vi "Update VI Properties.vi"() -> ()   [LabVIEW 2013, in "update vi properties.lvlib"]
uses:
  update vi properties.lvlib
  user action.ctl
  Event Data.ctl
  <vilib>/picture/picture.llb/imagedata.ctl
panel:
  in  "Prompt?":bool
  in  "Adjust all?":bool
  in  "Load":bool
  in  "Error in":errorcluster
  in  "Event Data":T1
  in  "Controls":string[][](table)
  in  "Indicators":string[][](table)
  in  "Help Tag":string
  in  "Help Path":string
  out "Path to VI":string
  in  "VI Description":string
  out "VI Conn Pane":picture
  in  "Select a VI to View/Edit Properties:":i32(listbox)=-1
  in  "Action":T2
  in  "OK":bool
  in  "Cancel":bool
  in  "Apply":bool
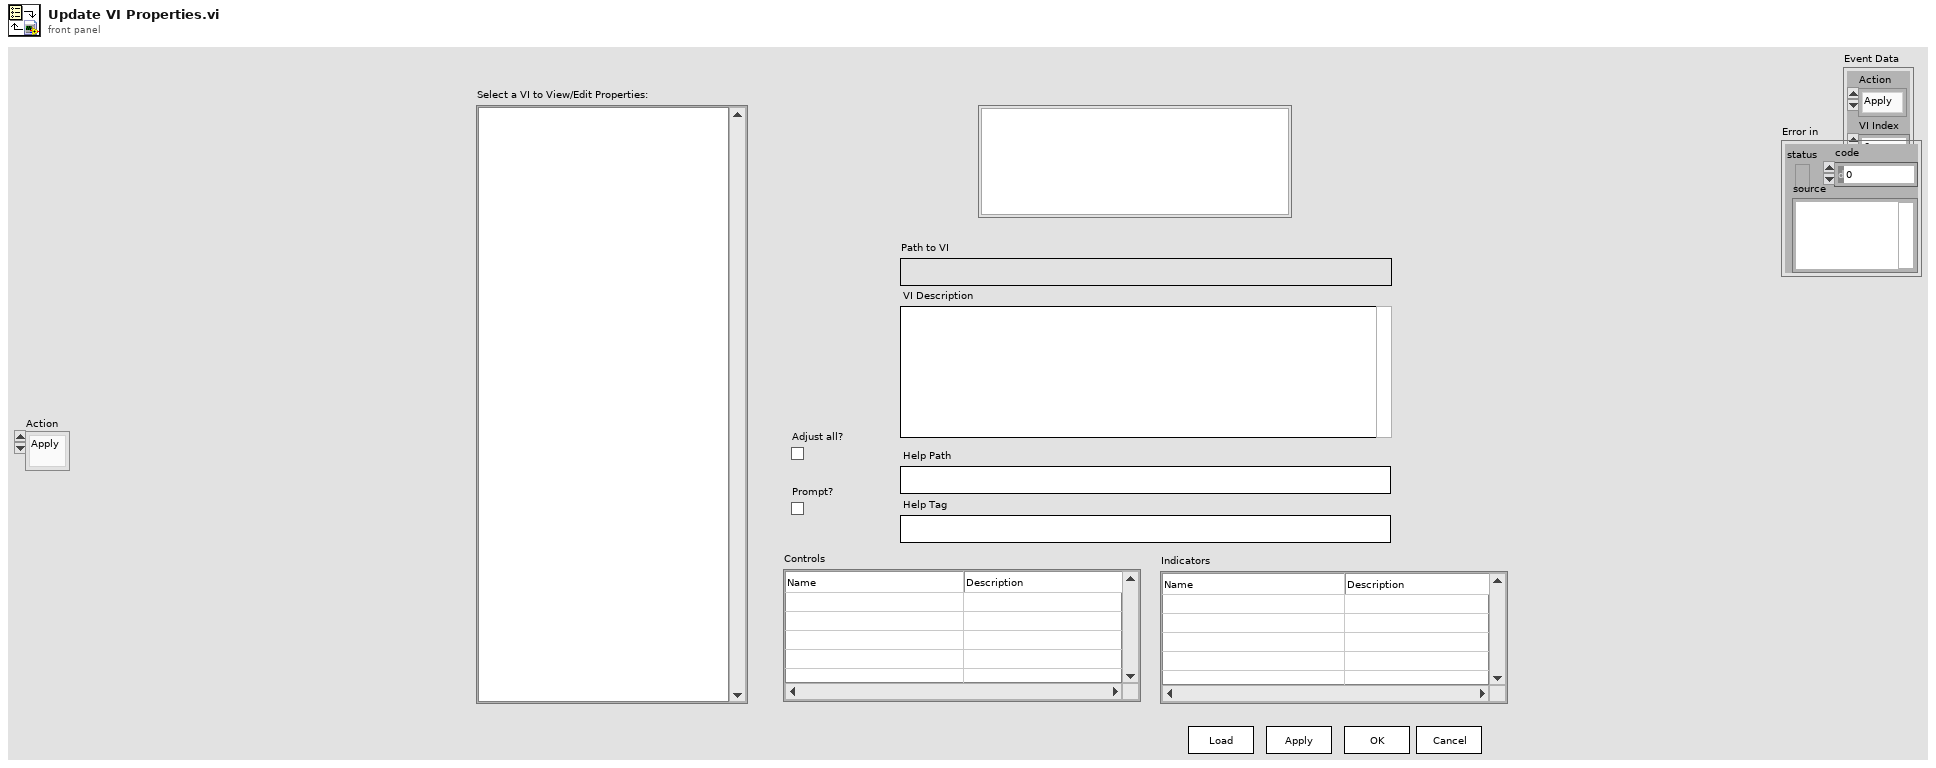
[diagram p1: front panel]
types:
  T1 = typedef "update vi properties.lvlib/Event Data.ctl" = cluster{"Action":T2, "VI Index":i32}
  T2 = typedef "update vi properties.lvlib/user action.ctl" = enum16{"Apply", "Cancel", "VI Selected", "Value Changed", "Load VIs"}
  T3 = typedef "imagedata.ctl" = cluster{"image type":i32, "image depth":i32, "image":u8[], "mask":u8[], "colors":u32[], "Rectangle":cluster{"left":i16, "top":i16, "right":i16, "bottom":i16}}
  T4 = enum32{"invalid VI type", "Standard VI", "Control VI", "Global VI", "Polymorphic VI", "Configuration VI", "SubSystem", "Facade VI", "Method VI", "Statechart Diagram VI"}[]
  T5 = enum32{"invalid VI type", "Standard VI", "Control VI", "Global VI", "Polymorphic VI", "Configuration VI", "SubSystem", "Facade VI", "Method VI", "Statechart Diagram VI"}
  T6 = enum8{"Enabled", "Disabled", "Disabled and Grayed Out"}
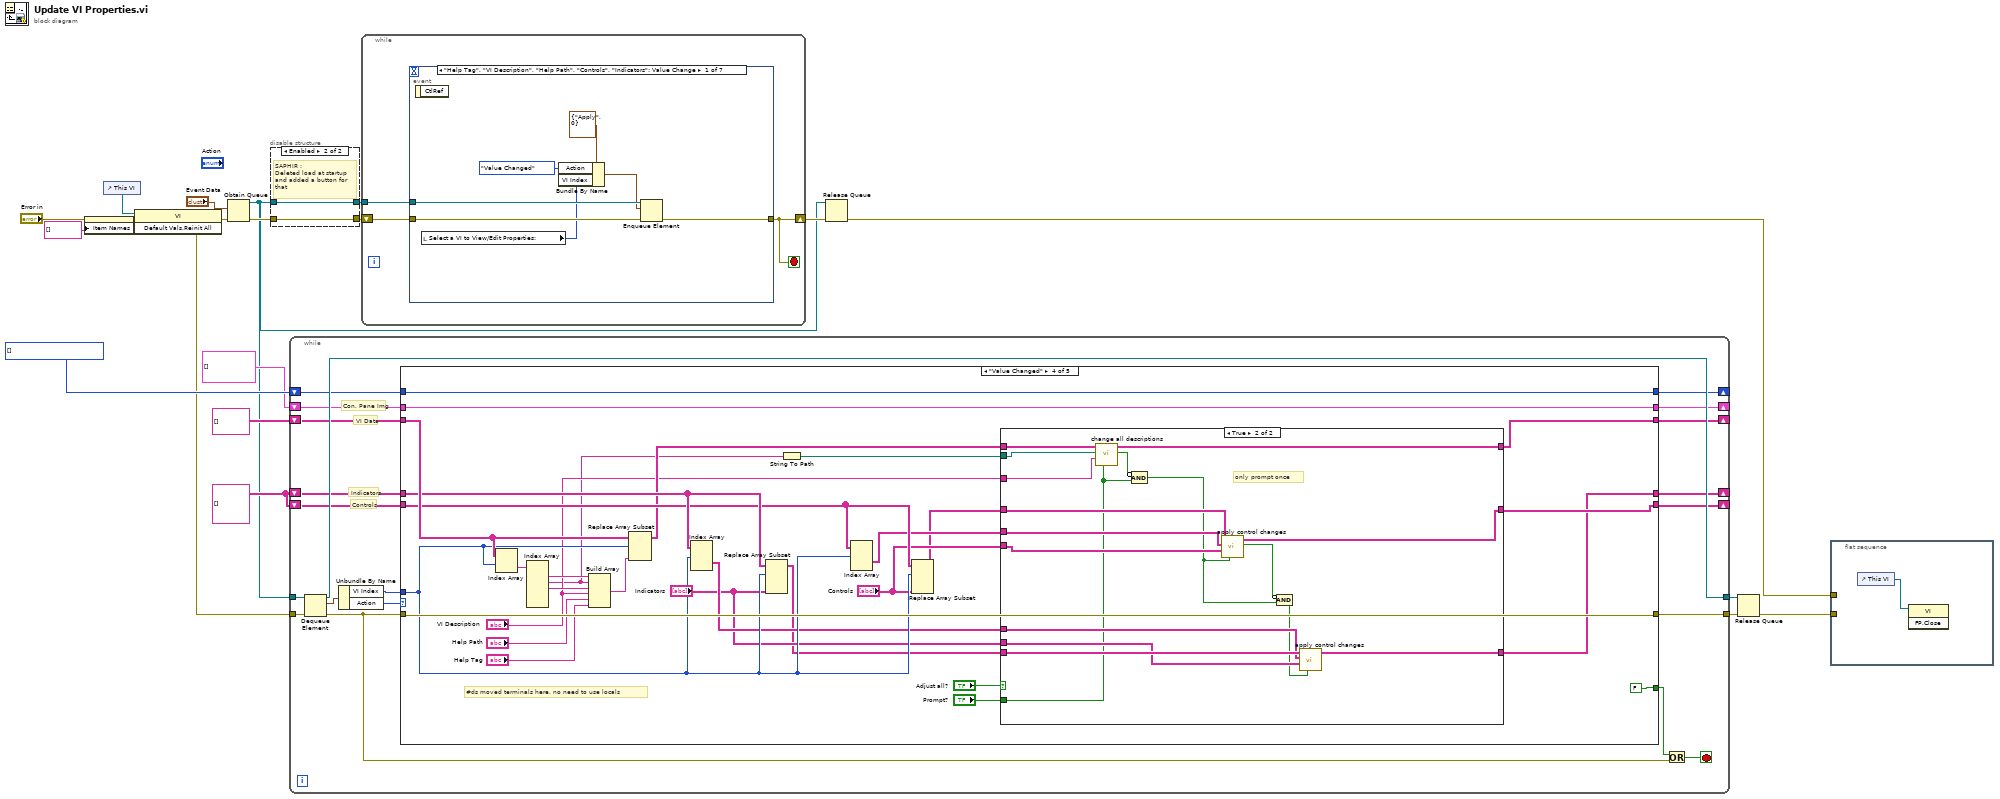
[diagram p0: block diagram]
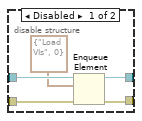
[diagram p2: hidden frame]
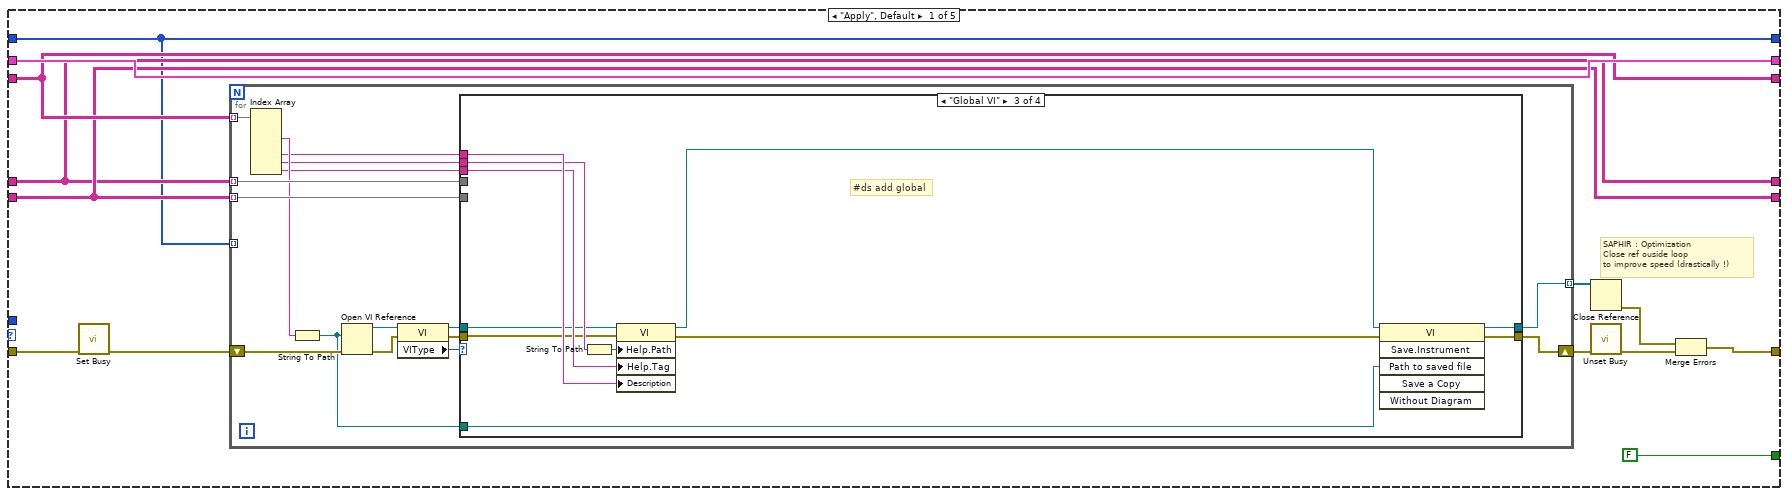
[diagram p3: hidden frame]
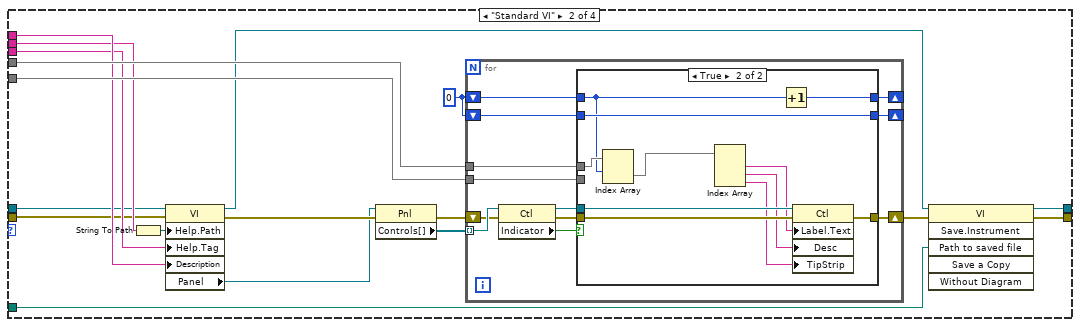
[diagram p5: hidden frame]
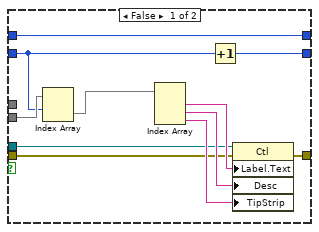
[diagram p6: hidden frame]
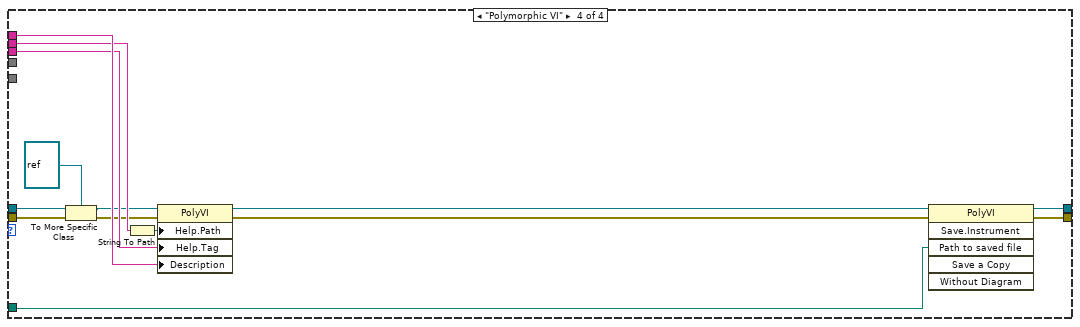
[diagram p7: hidden frame]
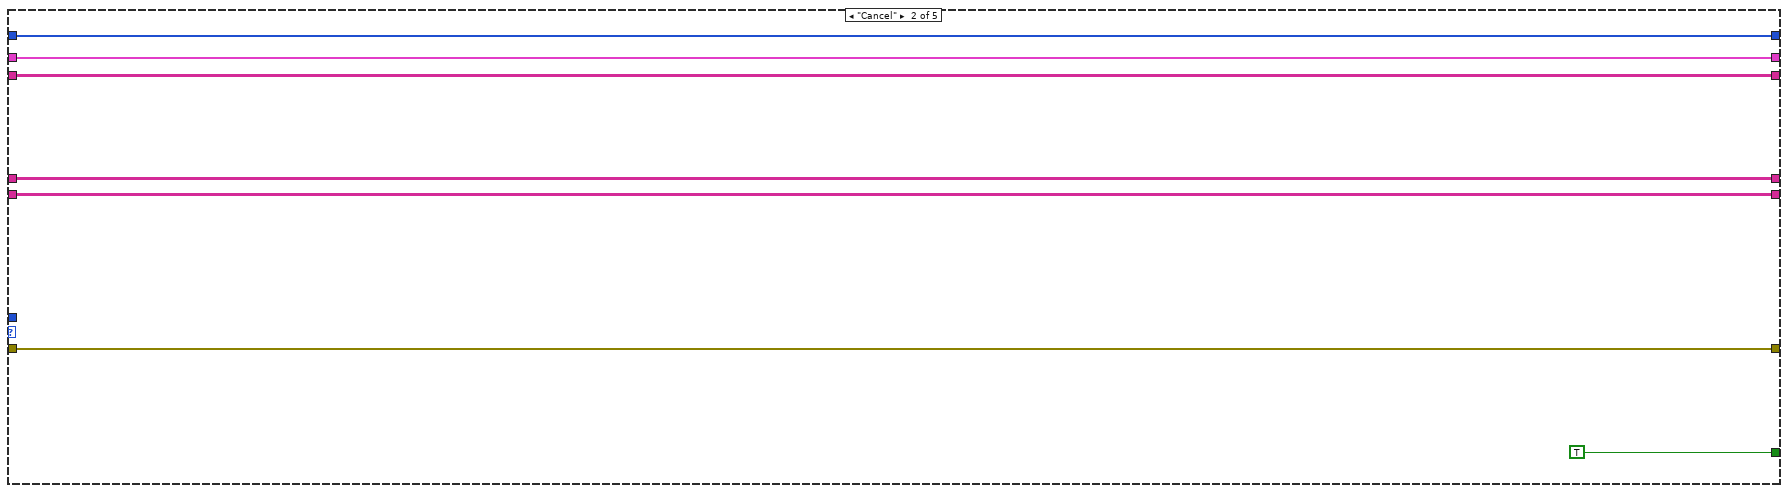
[diagram p8: hidden frame]
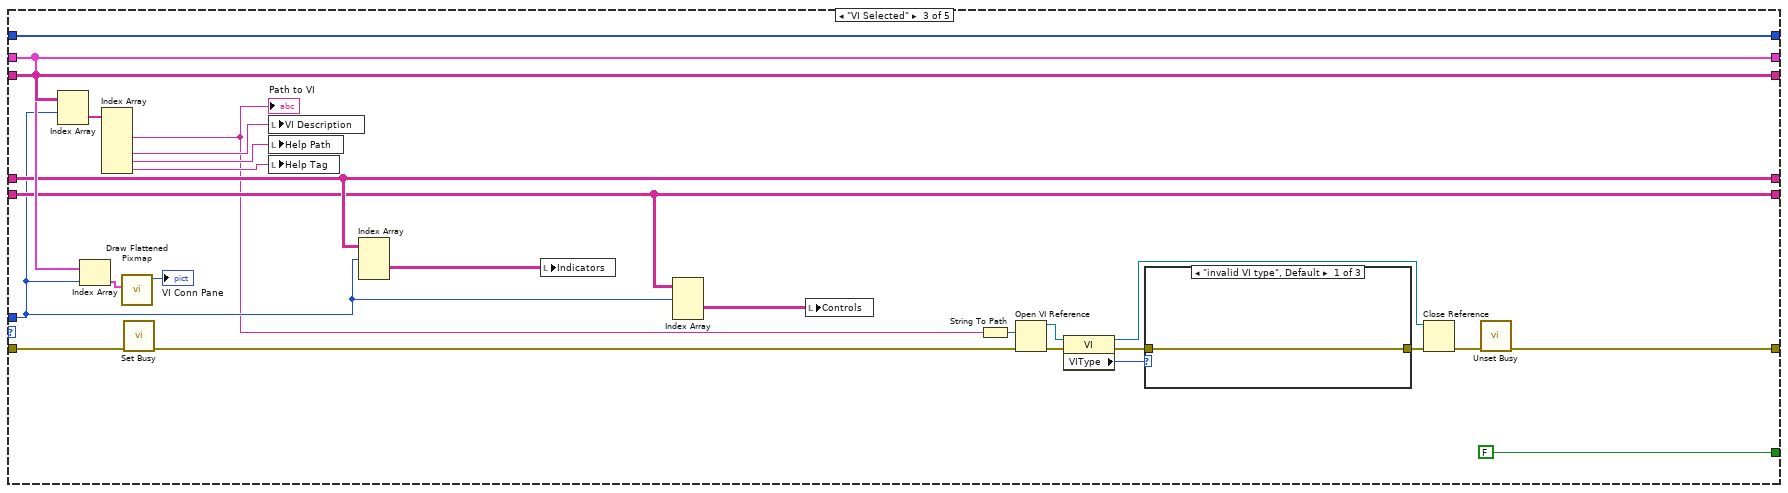
[diagram p9: hidden frame]
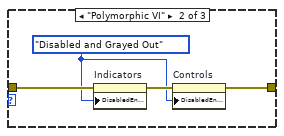
[diagram p10: hidden frame]
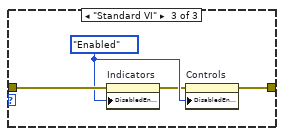
[diagram p11: hidden frame]
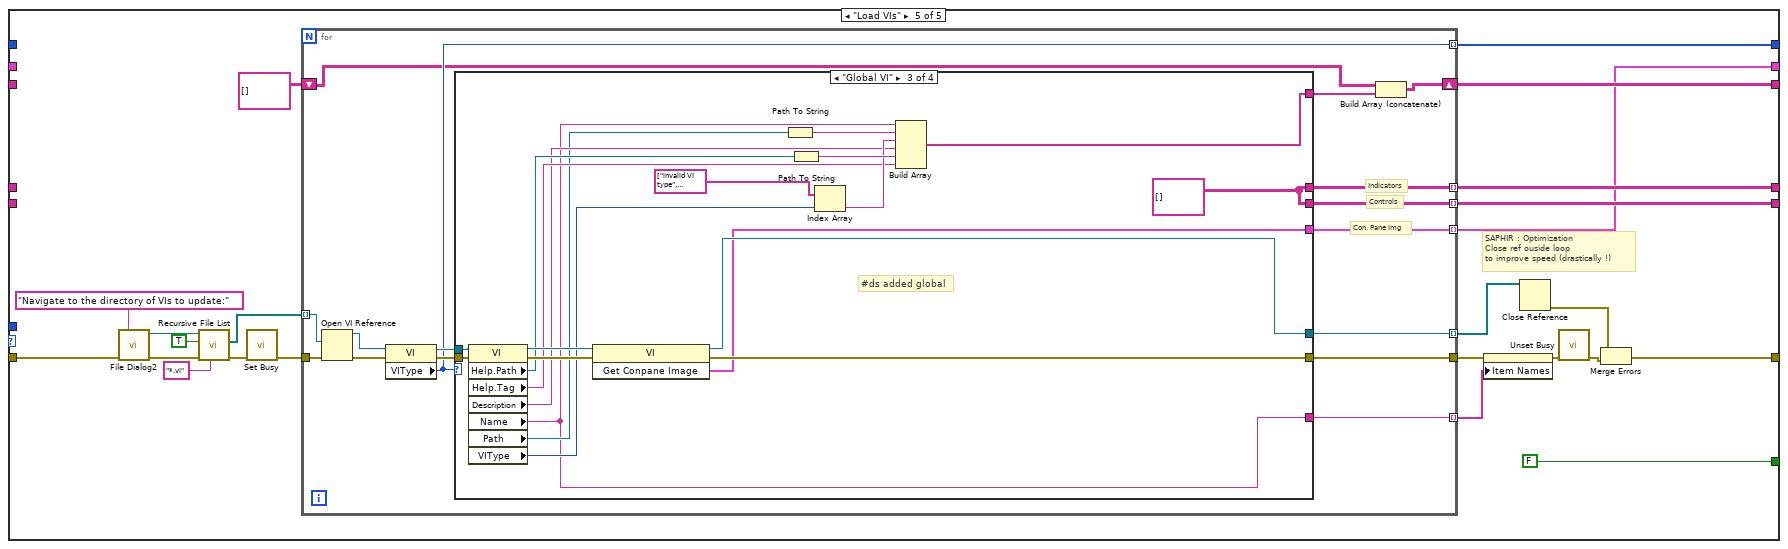
[diagram p13: hidden frame]
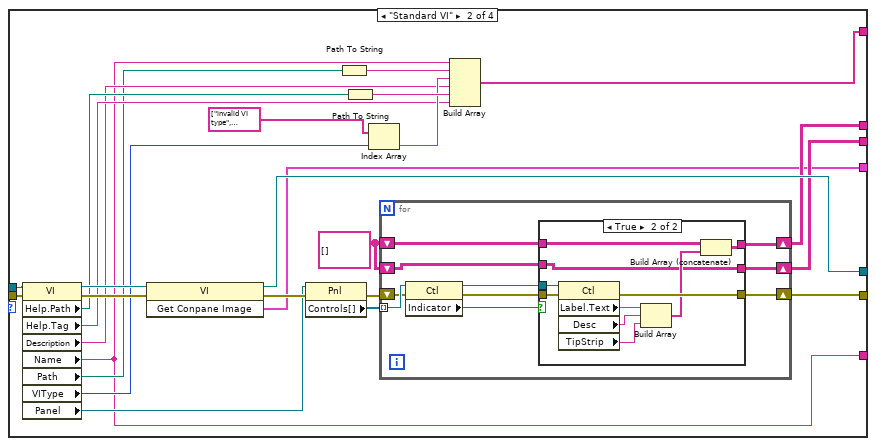
[diagram p15: hidden frame]
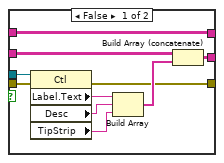
[diagram p16: hidden frame]
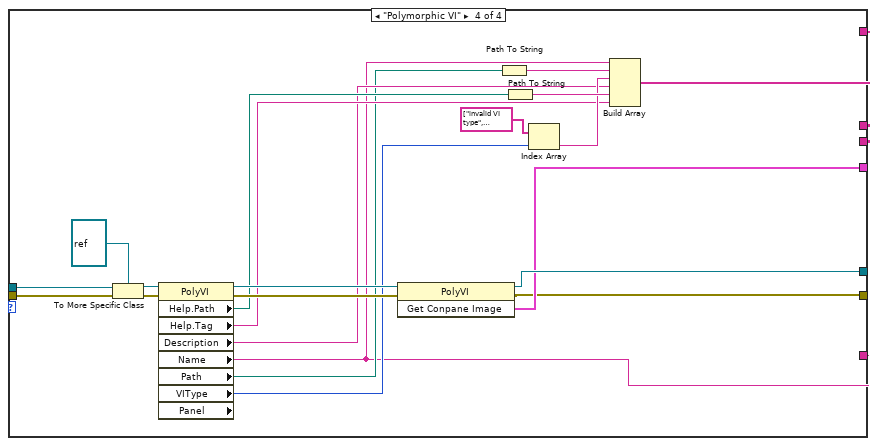
[diagram p17: hidden frame]
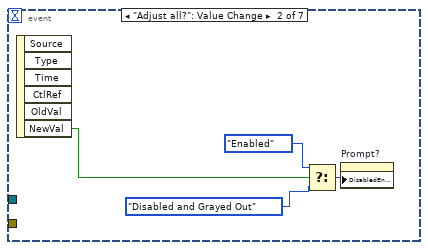
[diagram p18: hidden frame]
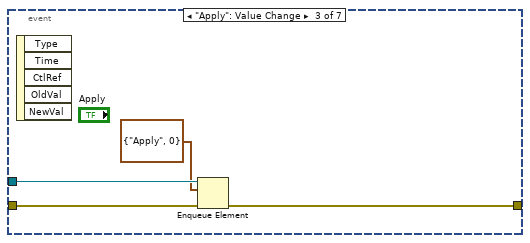
[diagram p19: hidden frame]
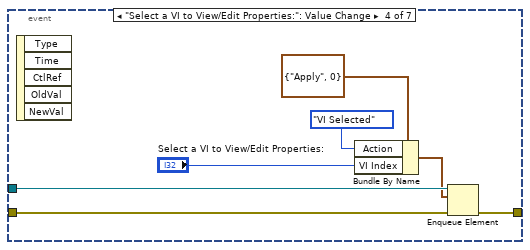
[diagram p20: hidden frame]
diagram:
  w11 = string[][][] []
  w13 = T4 [] items=["invalid VI type", "Standard VI", "Control VI", "Global VI", "Polymorphic VI", "Configuration VI", "SubSystem", "Facade VI", "Method VI", "Statechart Diagram VI"]
  n1 = property on="Select a VI to View/Edit Properties:" class="LstBox (strict)"(error in="Error in", "Item Names"=string[] []) -> (error out=w6:errorcluster)  [unwired: 1 in, 1 out]
  n2 = control-ref of="This VI"() -> (w9:refnum<vi>)
  n3 = invoke class="VI" method="Default Vals.Reinit All"(reference=w9, error in=w6) -> (error out=w8:errorcluster)  [unwired: 1 in, 2 out]
  n4 = Obtain Queue(element data type="Event Data", error in (no error)=w8) -> (queue out=w3:refnum<queue>, error out=w16:errorcluster)  [unwired: 3 in, 1 out]
  n5 = disable-structure shown="Enabled" {
    disable-tunnel: w16 -> [w24 w26]
    disable-tunnel: [w23 w26] -> w15
    disable-tunnel: w3 -> [w22 w25]
    disable-tunnel: [w21 w25] -> w14
    frame Disabled {
      n6 = Enqueue Element(queue=w22, element=T1 {"Action"=enum."Load VIs", "VI Index"=0}, error in (no error)=w24) -> (queue out=w21:refnum<queue>, error out=w23:errorcluster)  [unwired: 1 in, 1 out]
    }
    frame Enabled {
      # "SAPHIR :\nDeleted load at startup\nand added a button for\nthat"
    }
  }
  n7 = while {
    tunnel: w8 -> [w34]
    tunnel: w3 -> [w46]
    tunnel: [w31] -> w19
    tunnel: [w45] -> w18
    shift-right: [w38] -> _
    shift-left: string[][] [] -> [w39]
    shift-right: [w35] -> _
    shift-left: T3[] [] -> [w40]
    shift-right: [w37] -> _
    shift-left: w11 -> [w41]
    shift-right: [w36] -> _
    shift-left: w11 -> [w42]
    shift-right: [w32] -> _
    shift-left: w13 -> [w33]
    stop <- w28 stop-if-true
    # "VI Data"
    # "Controls"
    # "Indicators"
    # "Con. Pane Img"
    n8 = Dequeue Element(queue=w46, error in (no error)=w34) -> (queue out=w45:refnum<queue>, element=w44:T1, error out=w29:errorcluster)  [unwired: 1 in, 1 out]
    n9 = Unbundle By Name(w44) -> ("VI Index"=w43:i32, "Action"=w30:T2)
    n10 = case shown="\"Value Changed\"" w30 {
      tunnel: w29 -> [w58 w160 w180 w225 w265]
      tunnel: [FALSE TRUE FALSE FALSE FALSE] -> w27
      tunnel: [w48 w160 w162 w225 w247] -> w31
      tunnel: w43 -> [_ _ w176 w213 _]
      tunnel: w42 -> [w55 w157 w177 w214 _]
      tunnel: w41 -> [w54 w158 w178 w215 _]
      tunnel: w40 -> [w57 w156 w185 w224 _]
      tunnel: w39 -> [w56 w159 w186 w219 _]
      tunnel: [w56 w159 w186 w202 w259] -> w38
      tunnel: [w54 w158 w178 w204 w256] -> w37
      tunnel: [w55 w157 w177 w205 w255] -> w36
      tunnel: [w57 w156 w185 w224 w254] -> w35
      tunnel: w33 -> [w53 w155 w173 w218 _]
      tunnel: [w53 w155 w173 w218 w258] -> w32
      frame "Apply", Default {
        # "SAPHIR : Optimization\nClose ref ouside loop\nto improve speed (drastically !)"
        n11 = call <vilib>:"Set Busy.vi"("error in (no error)"=w58) -> ("error out"=w52:errorcluster)  [unwired: 9 in, 1 out]
        n12 = for {
          shift-right: [w61] -> w51
          shift-left: w52 -> [w74]
          tunnel: w56 -> [w75] mode=indexing
          tunnel: w55 -> [w72] mode=indexing
          tunnel: w54 -> [w73] mode=indexing
          tunnel: w53 -> [_] mode=indexing
          tunnel: [w60] -> w49 mode=indexing
          n13 = Index Array(array=w75) -> (element #2=w71:string, element #4=w70:string, element #5=w68:string, element #6=w69:string)  [unwired: 6 in, 2 out]
          n14 = String To Path(string=w71) -> (path=w67:path)
          n15 = Open VI Reference(vi path=w67, error in (no error)=w74) -> (vi reference=w66:refnum<vi>, error out=w63:errorcluster)  [unwired: 4 in]
          n16 = property class="VI"(reference=w66, error in=w63) -> (reference out=w65:refnum<vi>, error out=w64:errorcluster, "VIType"=w62:T5)
          n17 = case shown="\"Global VI\"" w62 {
            tunnel: [w76 w95 w140 w154] -> w60
            tunnel: [w77 w94 w139 w153] -> w61
            tunnel: w73 -> [_ w93 _ _]
            tunnel: w72 -> [_ w92 _ _]
            tunnel: w65 -> [w76 w79 w131 w146]
            tunnel: w64 -> [w77 w78 w130 w145]
            tunnel: w70 -> [_ w91 w138 w152]
            tunnel: w69 -> [_ w90 w137 w151]
            tunnel: w68 -> [_ w88 w135 w149]
            tunnel: w67 -> [_ w87 w134 w148]
            frame "invalid VI type", Default {
            }
            frame "Standard VI" {
              w80 = 0
              n18 = String To Path(string=w88) -> (path=w89:path)
              n19 = property class="VI"(reference=w79, error in=w78, "Help.Path"=w89, "Help.Tag"=w90, "Description"=w91) -> (reference out=w83:refnum<vi>, error out=w86:errorcluster, "Panel"=w85:refnum<vi>)
              n20 = property class="Pnl"(reference=w85, error in=w86) -> (error out=w81:errorcluster, "Controls[]"=w82:refnum<vi>[])  [unwired: 1 out]
              n21 = for {
                tunnel: w82 -> [w107] mode=indexing
                shift-right: [w96] -> w84
                shift-left: w81 -> [w106]
                tunnel: w93 -> [w99]
                tunnel: w92 -> [w98]
                shift-right: [w101] -> _
                shift-left: w80 -> [w103]
                shift-right: [w100] -> _
                shift-left: w80 -> [w102]
                n22 = property class="Ctl"(reference=w107, error in=w106) -> (reference out=w97:refnum<vi>, error out=w104:errorcluster, "Indicator"=w105:bool)
                n23 = case shown="True" w105 {
                  tunnel: w104 -> [w109 w123]
                  tunnel: w103 -> [w117 w126]
                  tunnel: w102 -> [w108 w128]
                  tunnel: [w117 w129] -> w101
                  tunnel: [w118 w128] -> w100
                  tunnel: w99 -> [_ w127]
                  tunnel: w98 -> [w112 _]
                  tunnel: w97 -> [w110 w124]
                  tunnel: [w113 w122] -> w96
                  frame False {
                    n24 = Index Array(array=w112, index (row)=w108) -> (element=w116:string[])  [unwired: 1 in]
                    n25 = Index Array(array=w116) -> (element #1=w115:string, element #2=w114:string, element #3=w111:string)  [unwired: 3 in]
                    n26 = Increment(x=w108) -> (x+1=w118:i32)
                    n27 = property class="Ctl"(reference=w110, error in=w109, "Label.Text"=w115, "Desc"=w114, "TipStrip"=w111) -> (error out=w113:errorcluster)  [unwired: 1 out]
                  }
                  frame True {
                    n28 = Index Array(array=w127, index (row)=w126) -> (element=w125:string[])  [unwired: 1 in]
                    n29 = Index Array(array=w125) -> (element #1=w121:string, element #2=w120:string, element #3=w119:string)  [unwired: 3 in]
                    n30 = Increment(x=w126) -> (x+1=w129:i32)
                    n31 = property class="Ctl"(reference=w124, error in=w123, "Label.Text"=w121, "Desc"=w120, "TipStrip"=w119) -> (error out=w122:errorcluster)  [unwired: 1 out]
                  }
                }
              }
              n32 = invoke class="VI" method="Save.Instrument"(reference=w83, error in=w84, "Path to saved file"=w87) -> (reference out=w95:refnum<vi>, error out=w94:errorcluster)  [unwired: 3 in, 4 out]
            }
            frame "Global VI" {
              # "#ds add global"
              n33 = String To Path(string=w135) -> (path=w136:path)
              n34 = property class="VI"(reference=w131, error in=w130, "Help.Path"=w136, "Help.Tag"=w137, "Description"=w138) -> (reference out=w132:refnum<vi>, error out=w133:errorcluster)
              n35 = invoke class="VI" method="Save.Instrument"(reference=w132, error in=w133, "Path to saved file"=w134) -> (reference out=w140:refnum<vi>, error out=w139:errorcluster)  [unwired: 3 in, 4 out]
            }
            frame "Polymorphic VI" {
              n36 = To More Specific Class(target class=refnum<vi> refnum, reference=w146, error in=w145) -> (specific class reference=w144:refnum<vi>, error out=w143:errorcluster)
              n37 = String To Path(string=w149) -> (path=w150:path)
              n38 = property class="PolyVI"(reference=w144, error in=w143, "Help.Path"=w150, "Help.Tag"=w151, "Description"=w152) -> (reference out=w142:refnum<vi>, error out=w141:errorcluster)
              n39 = invoke class="PolyVI" method="Save.Instrument"(reference=w142, error in=w141, "Path to saved file"=w148) -> (reference out=w154:refnum<vi>, error out=w153:errorcluster)  [unwired: 3 in, 4 out]
            }
          }
        }
        n40 = Close Reference(reference=w49) -> (error out=w47:errorcluster)  [unwired: 1 in]
        n41 = call <vilib>:"Unset Busy.vi"("error in (no error)"=w51) -> ("error out"=w50:errorcluster)  [unwired: 10 in]
        n42 = Merge Errors(w47, w50) -> (w48:errorcluster)
      }
      frame "Cancel" {
      }
      frame "VI Selected" {
        n43 = Index Array(array=w186, index (row)=w176) -> (element=w184:string[])  [unwired: 1 in]
        n44 = Index Array(array=w185, index=w176) -> (element=w187:T3)
        n45 = Index Array(array=w184) -> (element #2=w172:string, element #4=w183:string, element #5=w182:string, element #6=w181:string)  [unwired: 6 in, 2 out]
        "Path to VI" <- w172
        n46 = call <vilib>:"Draw Flattened Pixmap.vi"("image data"=w187) -> ("new picture"=→"VI Conn Pane":picture)  [unwired: 8 in]
        n47 = call <vilib>:"Set Busy.vi"("error in (no error)"=w180) -> ("error out"=w163:errorcluster)  [unwired: 9 in, 1 out]
        n48 = local write "VI Description"(w183) -> ()
        n49 = local write "Help Path"(w182) -> ()
        n50 = local write "Help Tag"(w181) -> ()
        n51 = Index Array(array=w178, index (dim 0)=w176) -> (element=w174:string[][])  [unwired: 2 in]
        n52 = local write "Indicators"(w174) -> ()
        n53 = Index Array(array=w177, index (dim 0)=w176) -> (element=w175:string[][])  [unwired: 2 in]
        n54 = local write "Controls"(w175) -> ()
        n55 = String To Path(string=w172) -> (path=w171:path)
        n56 = Open VI Reference(vi path=w171, error in (no error)=w163) -> (vi reference=w170:refnum<vi>, error out=w169:errorcluster)  [unwired: 4 in]
        n57 = property class="VI"(reference=w170, error in=w169) -> (reference out=w164:refnum<vi>, error out=w167:errorcluster, "VIType"=w168:T5)
        n58 = case shown="\"invalid VI type\", Default" w168 {
          tunnel: w167 -> [w189 w192 w197]
          tunnel: [w189 w191 w194] -> w166
          frame "invalid VI type", Default {
          }
          frame "Polymorphic VI" {
            w190 = T6."Disabled and Grayed Out" ("Disabled")
            n59 = property on="Indicators" class="Tbl (strict)"(error in=w192, "DisabledEnum"=w190) -> (error out=w193:errorcluster)  [unwired: 1 in, 1 out]
            n60 = property on="Controls" class="Tbl (strict)"(error in=w193, "DisabledEnum"=w190) -> (error out=w191:errorcluster)  [unwired: 1 in, 1 out]
          }
          frame "Standard VI" {
            w196 = T6."Enabled" ("Disabled")
            n61 = property on="Indicators" class="Tbl (strict)"(error in=w197, "DisabledEnum"=w196) -> (error out=w195:errorcluster)  [unwired: 1 in, 1 out]
            n62 = property on="Controls" class="Tbl (strict)"(error in=w195, "DisabledEnum"=w196) -> (error out=w194:errorcluster)  [unwired: 1 in, 1 out]
          }
        }
        n63 = Close Reference(reference=w164, error in (no error)=w166) -> (error out=w165:errorcluster)
        n64 = call <vilib>:"Unset Busy.vi"("error in (no error)"=w165) -> ("error out"=w162:errorcluster)  [unwired: 10 in]
      }
      frame "Value Changed" {
        # "#ds moved terminals here, no need to use locals"
        n65 = Index Array(array=w219, index (row)=w213) -> (element=w223:string[])  [unwired: 1 in]
        n66 = Index Array(array=w223) -> (element #1=w222:string, element #2=w199:string, element #3=w221:string)  [unwired: 6 in, 3 out]
        n67 = Build Array(w222, w199, w221, "VI Description", "Help Path", "Help Tag") -> (w220:string[])
        n68 = Replace Array Subset(array=w219, new element=w220, index (row)=w213) -> (w201:string[][])  [unwired: 1 in]
        n69 = Index Array(array=w215, index (dim 0)=w213) -> (element=w208:string[][])  [unwired: 2 in]
        n70 = Replace Array Subset(array=w215, new element="Indicators", index (dim 0)=w213) -> (w203:string[][][])  [unwired: 2 in]
        n71 = String To Path(string=w199) -> (path=w198:path)
        n72 = Index Array(array=w214, index (dim 0)=w213) -> (element=w209:string[][])  [unwired: 2 in]
        n73 = Replace Array Subset(array=w214, new element="Controls", index (dim 0)=w213) -> (w206:string[][][])  [unwired: 2 in]
        n74 = case shown="True" "Adjust all?" {
          tunnel: "Prompt?" -> [_ w234]
          tunnel: "Controls" -> [_ w240]
          tunnel: w209 -> [_ w241]
          tunnel: w208 -> [_ w238]
          tunnel: "Indicators" -> [_ w237]
          tunnel: w206 -> [w229 w243]
          tunnel: [w229 w242] -> w205
          tunnel: w203 -> [w228 w239]
          tunnel: [w228 w236] -> w204
          tunnel: [w227 w246] -> w202
          tunnel: w201 -> [w227 w245]
          tunnel: "VI Description" -> [_ w235]
          tunnel: w198 -> [_ w244]
          frame False {
          }
          frame True {
            # "only prompt once"
            n75 = call "change all descriptions.vi"("Prompt?"=w234, "new"=w235, "Path"=w244, "dataset in"=w245) -> ("adjust all"=w233:bool, "dataset out"=w246:string[][])  [unwired: 6 in]
            n76 = Compound Arithmetic op=AND(invert w233, w234) -> (w231:bool)
            n77 = call "apply control changes.vi"("Prompt?"=w231, "new"=w240, "old"=w241, "dataset in"=w243) -> ("adjust all?"=w232:bool, "dataset out"=w242:string[][][])  [unwired: 6 in]
            n78 = Compound Arithmetic op=AND(invert w232, w231) -> (w230:bool)
            n79 = call "apply control changes.vi"("Prompt?"=w230, "new"=w237, "old"=w238, "dataset in"=w239) -> ("dataset out"=w236:string[][][])  [unwired: 6 in, 1 out]
          }
        }
      }
      frame "Load VIs" {
        # "SAPHIR : Optimization\nClose ref ouside loop\nto improve speed (drastically !)"
        n80 = call "File Dialog2"("prompt"="Navigate to the directory of VIs to update:", "error in"=w265) -> ("selected path"=w267:path, "error out"=w268:errorcluster)  [unwired: 10 in, 2 out]
        n81 = call <vilib>:"Recursive File List.vi"("pattern"="*.vi", "error in (no error)"=w268, "Treat LLBs as Folders?"=TRUE, "Folder Path"=w267) -> ("error out"=w263:errorcluster, "All Files in Dir"=w261:path[])  [unwired: 3 in, 3 out]
        n82 = call <vilib>:"Set Busy.vi"("error in (no error)"=w263) -> ("error out"=w262:errorcluster)  [unwired: 9 in, 1 out]
        n83 = for {
          tunnel: w262 -> [w283]
          tunnel: w261 -> [w282] mode=indexing
          shift-right: [w276] -> w259
          shift-left: string[][] [] -> [w278]
          tunnel: [w279] -> w258 mode=indexing
          tunnel: [w275] -> w257 mode=indexing
          tunnel: [w274] -> w256 mode=indexing
          tunnel: [w273] -> w255 mode=indexing
          tunnel: [w272] -> w254 mode=indexing
          tunnel: [w271] -> w253
          tunnel: [w270] -> w250 mode=indexing
          # "Controls"
          # "Indicators"
          # "Con. Pane Img"
          n84 = Open VI Reference(vi path=w282, error in (no error)=w283) -> (vi reference=w285:refnum<vi>, error out=w284:errorcluster)  [unwired: 4 in]
          n85 = property class="VI"(reference=w285, error in=w284) -> (reference out=w280:refnum<vi>, error out=w281:errorcluster, "VIType"=w279:T5)
          n86 = case shown="\"Global VI\"" w279 {
            tunnel: w281 -> [w287 w316 w365 w371]
            tunnel: w280 -> [w286 w315 w364 w369]
            tunnel: [string[] ["Invalid VI type"] w297 w349 w374] -> w277
            tunnel: ["" ("Name") w296 w348 w373] -> w275
            tunnel: [w289 w309 w347 w366] -> w274
            tunnel: [w289 w308 w347 w366] -> w273
            tunnel: [T3 {"image type"=0, "image depth"=0, "image"=[], "mask"=[], "colors"=[], "Rectangle"={"left"=0, "top"=0, "right"=0, "bottom"=0}} ("Get Conpane Image") w307 w359 w384] -> w272
            tunnel: [w287 w295 w361 w367] -> w271
            tunnel: [w286 w310 w360 w385] -> w270
            frame "invalid VI type", Default {
              w289 = string[][] []
            }
            frame "Standard VI" {
              w292 = string[][] []
              n87 = property class="VI"(reference=w315, error in=w316) -> (reference out=w314:refnum<vi>, error out=w313:errorcluster, "Help.Path"=w302:path, "Help.Tag"=w301:string, "Description"=w300:string, "Name"=w296:string, "Path"=w299:path, "VIType"=w298:T5, "Panel"=w311:refnum<vi>)
              n88 = invoke class="VI" method="Get Conpane Image"(reference=w314, error in=w313) -> (reference out=w310:refnum<vi>, error out=w312:errorcluster, "Get Conpane Image"=w307:T3)  [unwired: 1 in]
              n89 = property class="Pnl"(reference=w311, error in=w312) -> (error out=w293:errorcluster, "Controls[]"=w294:refnum<vi>[])  [unwired: 1 out]
              n90 = Path To String(path=w299) -> (string=w304:string)
              n91 = Path To String(path=w302) -> (string=w306:string)
              n92 = Index Array(array=string[] ["invalid VI type", "Standard VI", "Control VI", "Global VI", "Polymorphic VI", "Configuration VI", "SubSystem", "Facade VI", "Method VI", "Statechart Diagram VI"] ("Strings []"), index=w298) -> (element=w305:string)
              n93 = for {
                tunnel: w294 -> [w326] mode=indexing
                shift-right: [w321] -> w295
                shift-left: w293 -> [w325]
                shift-right: [w320] -> w309
                shift-left: w292 -> [w319]
                shift-right: [w318] -> w308
                shift-left: w292 -> [w317]
                n94 = property class="Ctl"(reference=w326, error in=w325) -> (reference out=w323:refnum<vi>, error out=w322:errorcluster, "Indicator"=w324:bool)
                n95 = case shown="True" w324 {
                  tunnel: w323 -> [w331 w346]
                  tunnel: w322 -> [w332 w345]
                  tunnel: [w330 w344] -> w321
                  tunnel: [w327 w338] -> w320
                  tunnel: w319 -> [w327 w340]
                  tunnel: [w329 w337] -> w318
                  tunnel: w317 -> [w328 w337]
                  frame False {
                    n96 = property class="Ctl"(reference=w331, error in=w332) -> (error out=w330:errorcluster, "Label.Text"=w336:string, "Desc"=w335:string, "TipStrip"=w334:string)  [unwired: 1 out]
                    n97 = Build Array(w336, w335, w334) -> (w333:string[])
                    n98 = Build Array (concatenate)(w328, w333) -> (w329:string[][])
                  }
                  frame True {
                    n99 = property class="Ctl"(reference=w346, error in=w345) -> (error out=w344:errorcluster, "Label.Text"=w343:string, "Desc"=w342:string, "TipStrip"=w341:string)  [unwired: 1 out]
                    n100 = Build Array(w343, w342, w341) -> (w339:string[])
                    n101 = Build Array (concatenate)(w340, w339) -> (w338:string[][])
                  }
                }
              }
              n102 = Build Array(w296, w304, w305, w300, w306, w301) -> (w297:string[])
            }
            frame "Global VI" {
              w347 = string[][] []
              # "#ds added global"
              n103 = property class="VI"(reference=w364, error in=w365) -> (reference out=w363:refnum<vi>, error out=w362:errorcluster, "Help.Path"=w354:path, "Help.Tag"=w353:string, "Description"=w352:string, "Name"=w348:string, "Path"=w351:path, "VIType"=w350:T5)
              n104 = invoke class="VI" method="Get Conpane Image"(reference=w363, error in=w362) -> (reference out=w360:refnum<vi>, error out=w361:errorcluster, "Get Conpane Image"=w359:T3)  [unwired: 1 in]
              n105 = Path To String(path=w351) -> (string=w356:string)
              n106 = Path To String(path=w354) -> (string=w358:string)
              n107 = Index Array(array=string[] ["invalid VI type", "Standard VI", "Control VI", "Global VI", "Polymorphic VI", "Configuration VI", "SubSystem", "Facade VI", "Method VI", "Statechart Diagram VI"] ("Strings []"), index=w350) -> (element=w357:string)
              n108 = Build Array(w348, w356, w357, w352, w358, w353) -> (w349:string[])
            }
            frame "Polymorphic VI" {
              w366 = string[][] []
              n109 = To More Specific Class(target class=refnum<vi> refnum, reference=w369, error in=w371) -> (specific class reference=w368:refnum<vi>, error out=w370:errorcluster)
              n110 = property class="PolyVI" props=["Help.Path", "Help.Tag", "Description", "Name", "Path", "VIType", "Panel"](reference=w368, error in=w370) -> (reference out=w387:refnum<vi>, error out=w386:errorcluster, "Help.Path"=w379:path, "Help.Tag"=w378:string, "Description"=w377:string, "Name"=w373:string, "Path"=w376:path, "VIType"=w375:T5)  [unwired: 1 out]
              n111 = invoke class="PolyVI" method="Get Conpane Image"(reference=w387, error in=w386) -> (reference out=w385:refnum<vi>, error out=w367:errorcluster, "Get Conpane Image"=w384:T3)  [unwired: 1 in]
              n112 = Path To String(path=w376) -> (string=w381:string)
              n113 = Path To String(path=w379) -> (string=w383:string)
              n114 = Index Array(array=string[] ["invalid VI type", "Standard VI", "Control VI", "Global VI", "Polymorphic VI", "Configuration VI", "SubSystem", "Facade VI", "Method VI", "Statechart Diagram VI"] ("Strings []"), index=w375) -> (element=w382:string)
              n115 = Build Array(w373, w381, w382, w377, w383, w378) -> (w374:string[])
            }
          }
          n116 = Build Array (concatenate)(w278, w277) -> (w276:string[][])
        }
        n117 = property on="Select a VI to View/Edit Properties:" class="LstBox (strict)"(error in=w253, "Item Names"=w257) -> (error out=w251:errorcluster)  [unwired: 1 in, 1 out]
        n118 = Close Reference(reference=w250) -> (error out=w249:errorcluster)  [unwired: 1 in]
        n119 = call <vilib>:"Unset Busy.vi"("error in (no error)"=w251) -> ("error out"=w248:errorcluster)  [unwired: 10 in]
        n120 = Merge Errors(w249, w248) -> (w247:errorcluster)
      }
    }
    n121 = Or(x=w27, y=w29) -> (x .or. y?=w28:bool)
  }
  n122 = while {
    shift-right: [w388] -> w4
    shift-left: w15 -> [w389]
    tunnel: w14 -> [w390]
    stop <- w388 stop-if-true
    n123 = event shown="[0] \"Help Tag\", \"VI Description\", \"Help Path\", \"Controls\", \"Indicators\": Value Change" {
      selector: _ -> [_ _ _ _ _ _ _]
      dyn-events: _ -> [_ _ _ _ _ _ _]
      timeout: _ -> [_ _ _ _ _ _ _]
      tunnel: w390 -> [w397 _ w405 w412 w416 w422 w426]
      tunnel: w389 -> [w396 _ w404 w411 w415 w423 w425]
      tunnel: [w395 _ w403 w407 w414 w419 w424] -> w388
      event "Help Tag", "VI Description", "Help Path", "Controls", "Indicators": Value Change {
        n124 = event-data() -> ()  [unwired: 1 in, 1 out]
        n125 = local read "Select a VI to View/Edit Properties:"() -> (w392:i32)
        n126 = Bundle By Name(cluster=T1 {"Action"=enum."Apply", "VI Index"=0} ("element"), "Action"=user_action."Value Changed", "VI Index"=w392) -> (w391:T1)
        n127 = Enqueue Element(queue=w397, element=w391, error in (no error)=w396) -> (error out=w395:errorcluster)  [unwired: 1 in, 2 out]
      }
      event "Adjust all?": Value Change {
        n128 = event-data() -> ("NewVal"=w398:bool)  [unwired: 1 in, 5 out]
        n129 = Select(t=T6."Enabled" ("Disabled"), s=w398, f=T6."Disabled and Grayed Out" ("Disabled")) -> (s? t:f=w401:T6)
        n130 = property on="Prompt?" class="Bool (strict)"("DisabledEnum"=w401) -> ()  [unwired: 2 in, 2 out]
      }
      event "Apply": Value Change {
        n131 = event-data() -> ()  [unwired: 1 in, 5 out]
        n132 = Enqueue Element(queue=w405, element=T1 {"Action"=enum."Apply", "VI Index"=0}, error in (no error)=w404) -> (error out=w403:errorcluster)  [unwired: 1 in, 2 out]
      }
      event "Select a VI to View/Edit Properties:": Value Change {
        n133 = event-data() -> ()  [unwired: 1 in, 5 out]
        n134 = Bundle By Name(cluster=T1 {"Action"=enum."Apply", "VI Index"=0} ("element"), "Action"=user_action."VI Selected", "VI Index"="Select a VI to View/Edit Properties:") -> (w408:T1)
        n135 = Enqueue Element(queue=w412, element=w408, error in (no error)=w411) -> (error out=w407:errorcluster)  [unwired: 1 in, 2 out]
      }
      event "Cancel": Value Change {
        n136 = event-data() -> ()  [unwired: 1 in, 5 out]
        n137 = Enqueue Element(queue=w416, element=T1 {"Action"=enum."Cancel", "VI Index"=0}, error in (no error)=w415) -> (error out=w414:errorcluster)  [unwired: 1 in, 2 out]
      }
      event "OK": Value Change {
        (unwired) FALSE ("Cancel")
        n138 = event-data() -> ()  [unwired: 1 in, 5 out]
        n139 = Enqueue Element(queue=w422, element=T1 {"Action"=enum."Apply", "VI Index"=0}, error in (no error)=w423) -> (queue out=w420:refnum<queue>, error out=w421:errorcluster)  [unwired: 1 in, 1 out]
        n140 = Enqueue Element(queue=w420, element=T1 {"Action"=enum."Cancel", "VI Index"=0}, error in (no error)=w421) -> (error out=w419:errorcluster)  [unwired: 1 in, 2 out]
      }
      event "Load": Value Change {
        n141 = event-data() -> ()  [unwired: 1 in, 5 out]
        n142 = Enqueue Element(queue=w426, element=T1 {"Action"=enum."Load VIs", "VI Index"=0}, error in (no error)=w425) -> (error out=w424:errorcluster)  [unwired: 1 in, 2 out]
      }
    }
  }
  n143 = Release Queue(queue=w3, error in (no error)=w4) -> (error out=w1:errorcluster)  [unwired: 1 in, 2 out]
  n144 = Release Queue(queue=w18, error in (no error)=w19) -> (error out=w2:errorcluster)  [unwired: 1 in, 2 out]
  n145 = flat-sequence {
    tunnel: w2 -> [_]
    tunnel: w1 -> [_]
    frame #0 {
      n146 = control-ref of="This VI"() -> (w428:refnum<vi>)
      n147 = invoke class="VI" method="FP.Close"(reference=w428) -> ()  [unwired: 2 in, 3 out]
    }
  }
